vi "FindNodeAtIndex.vi"(8 "DOM document":refnum<k20>, 9 "New Node Name":string="Drive", 10 "Index":u32=13, 11 "XML String":string="\n<Sequential>\n      <Sequential>\n            <Sequential>\n                  <Hi/>\n            </Sequential>\n      </Sequential>\n      <Drive/>\n      <Sequential>\n            <Hello/>\n      </Sequential>\n</Sequential>") -> ()   [LabVIEW 2017]
uses:
  <vilib>/regexp/Match Regular Expression.xnode
  <resource>/objmgr/DOMUserDefRef.rc
  <vilib>/xml/NI_XML.lvlib
panel:
  out "XML":string
  out "submatch 1":string="Sequential"
  out "Insert as child not sibling":bool
  out "Index":i32=3
  out "Text.Selection:Start":u32=223
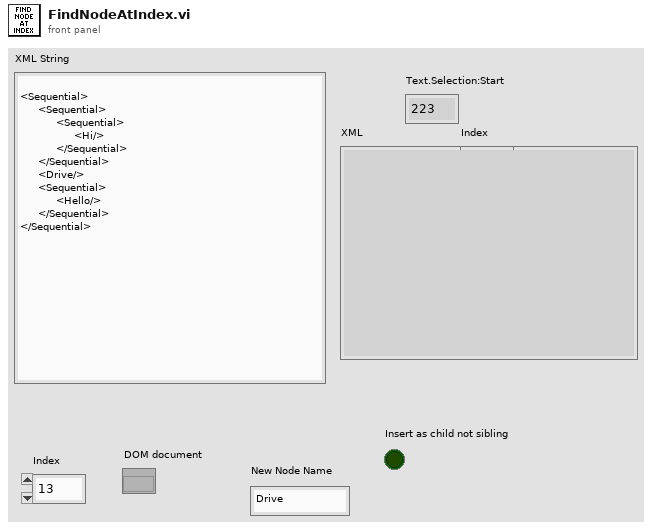
[diagram p1: front panel]
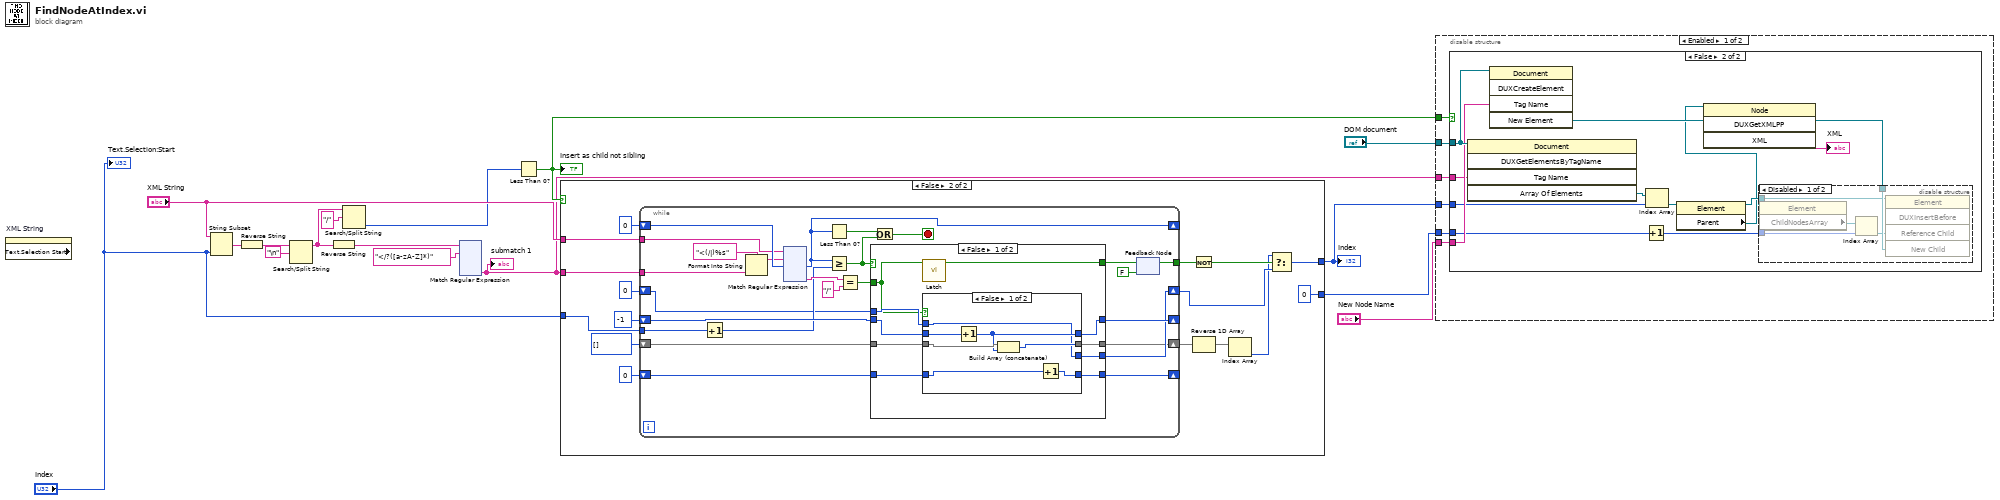
[diagram p0: block diagram]
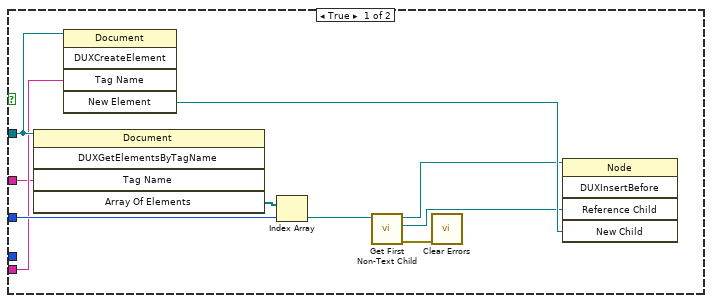
[diagram p2: hidden frame]
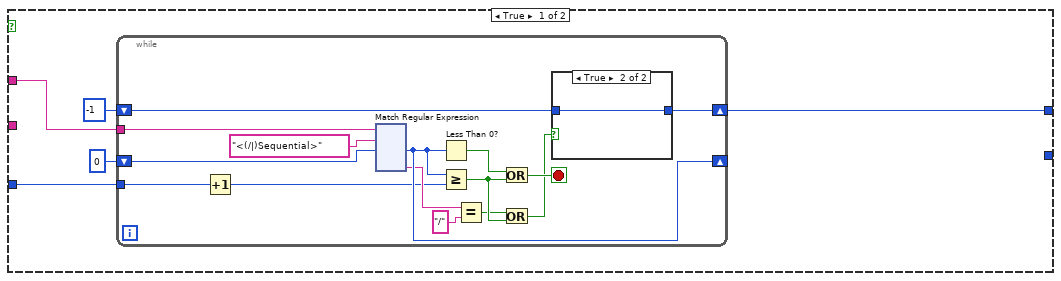
[diagram p5: hidden frame]
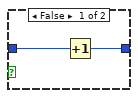
[diagram p6: hidden frame]
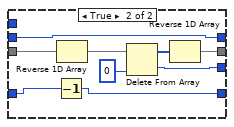
[diagram p7: hidden frame]
diagram:
  n1 = property on="XML String" class="Str" props=["Text", "Selection Start"]() -> ()  [unwired: 2 in, 3 out]
  n2 = String Subset(string="XML String", length (rest)="Index") -> (substring=w13:string)  [unwired: 1 in]
  n3 = Reverse String(1:w13) -> (0:w14:string)
  n4 = Search/Split String(string=w14, search string/char (-)="\n") -> (substring before match=w8:string)  [unwired: 1 in, 2 out]
  n5 = Reverse String(1:w8) -> (0:w10:string)
  n6 = Search/Split String(string=w8, search string/char (-)="/") -> (offset of match=w15:i32)  [unwired: 1 in, 2 out]
  n7 = xnode "Match Regular Expression"("input string"=w10, "regular expression"="</?([a-zA-Z]*)") -> ("submatch 1"=w2:string)  [unwired: 4 in, 5 out]
  "submatch 1" <- w2
  n8 = Less Than 0?(x=w15) -> (x < 0?=w5:bool)
  "Insert as child not sibling" <- w5
  n9 = case shown="False" w5 {
    tunnel: "XML String" -> [w21 w171]
    tunnel: [w18 w159] -> w7
    tunnel: "Index" -> [w17 w168]
    tunnel: [_ 0] -> w4
    tunnel: w2 -> [_ w164]
    frame True {
      n10 = while {
        tunnel: w21 -> [w26]
        shift-right: [w33] -> _
        shift-left: 0 -> [w35]
        tunnel: w17 -> [w25]
        shift-right: [w29] -> w18
        shift-left: -1 -> [w30]
        stop <- w28 stop-if-true
        n11 = Increment(x=w25) -> (x+1=w27:u32)
        n12 = xnode "Match Regular Expression"("input string"=w26, "regular expression"="<(/|)Sequential>", "offset (0)"=w35) -> ("offset past match"=w33:i32, "submatch 1"=w32:string)  [unwired: 3 in, 4 out]
        n13 = Less Than 0?(x=w33) -> (x < 0?=w34:bool)
        n14 = Greater Or Equal?(x=w33, y=w27) -> (x >= y?=w24:bool)
        n15 = Equal?(x=w32, y="/") -> (x = y?=w23:bool)
        n16 = Or(x=w34, y=w24) -> (x .or. y?=w28:bool)
        n17 = Or(x=w23, y=w24) -> (x .or. y?=w22:bool)
        n18 = case shown="True" w22 {
          tunnel: w30 -> [w37 w39]
          tunnel: [w38 w39] -> w29
          frame False {
            n19 = Increment(x=w37) -> (x+1=w38:i32)
          }
          frame True {
          }
        }
      }
    }
    frame False {
      n20 = while {
        tunnel: w171 -> [w188]
        shift-right: [w183] -> _
        shift-left: 0 -> [w196]
        tunnel: w168 -> [w187]
        shift-right: [w191] -> _
        shift-left: -1 -> [w192]
        shift-right: [w175] -> w158
        shift-left: i32[] [] -> [w182]
        shift-right: [w184] -> _
        shift-left: 0 -> [w186]
        tunnel: w164 -> [w180]
        shift-right: [w177] -> w161
        shift-left: 0 ("Numeric") -> [w176]
        tunnel: [w172] -> w162
        stop <- w190 stop-if-true
        n21 = Increment(x=w187) -> (x+1=w189:u32)
        n22 = Format Into String(format string="<(/|)%s" ("regular expression"), w180) -> (resulting string=w179:string)  [unwired: 2 in, 1 out]
        n23 = xnode "Match Regular Expression"("input string"=w188, "regular expression"=w179, "offset (0)"=w196) -> ("offset past match"=w183:i32, "submatch 1"=w194:string)  [unwired: 3 in, 4 out]
        n24 = Less Than 0?(x=w183) -> (x < 0?=w195:bool)
        n25 = Greater Or Equal?(x=w183, y=w189) -> (x >= y?=w185:bool)
        n26 = Equal?(x=w194, y="/") -> (x = y?=w178:bool)
        n27 = case shown="False" w185 {
          tunnel: w192 -> [w206 w226]
          tunnel: [w205 w226] -> w191
          tunnel: w186 -> [w204 w225]
          tunnel: w178 -> [w198 _]
          tunnel: [w199 w225] -> w184
          tunnel: w182 -> [w203 w224]
          tunnel: [w202 w224] -> w175
          tunnel: [w201 w223] -> w177
          tunnel: w176 -> [w200 w223]
          tunnel: [w197 _] -> w174
          frame False {
            n28 = call "Latch.vi"("Input"=w198) -> ("Output"=w197:bool)  [unwired: 10 in]
            n29 = case shown="False" w198 {
              tunnel: w206 -> [w211 w220]
              tunnel: [w210 w220] -> w205
              tunnel: w204 -> [w208 w215]
              tunnel: w203 -> [w213 w222]
              tunnel: [w212 w221] -> w202
              tunnel: [w209 w216] -> w201
              tunnel: w200 -> [w209 _]
              tunnel: [w207 w214] -> w199
              frame False {
                n30 = Increment(x=w211) -> (x+1=w210:i32)
                n31 = Build Array (concatenate)(w213, w210) -> (w212:i32[])
                n32 = Increment(x=w208) -> (x+1=w207:i32)
              }
              frame True {
                n33 = Decrement(x=w215) -> (x-1=w214:i32)
                n34 = Reverse 1D Array(array=w222) -> (reversed array=w219:i32[])
                n35 = Delete From Array(array=w219, index=0) -> (deleted portion=w216:i32, array with subset deleted=w217:i32[])  [unwired: 1 in]
                n36 = Reverse 1D Array(array=w217) -> (reversed array=w221:i32[])
              }
            }
          }
          frame True {
          }
        }
        n37 = Or(x=w195, y=w185) -> (x .or. y?=w190:bool)
        n38 = feedback-in #1(w174) -> ()
        n39 = feedback #1(FALSE ("Output")) -> (w172:bool)
      }
      n40 = Not(x=w162) -> (.not. x?=w160:bool)
      n41 = Reverse 1D Array(array=w158) -> (reversed array=w157:i32[])
      n42 = Index Array(array=w157) -> (element=w156:i32)  [unwired: 1 in]
      n43 = Select(t=w156, s=w160, f=w161) -> (s? t:f=w159:i32)
    }
  }
  "Index" <- w7
  n44 = disable-structure shown="Enabled" {
    disable-tunnel: "DOM document" -> [w348 _]
    disable-tunnel: w7 -> [w347 _]
    disable-tunnel: "New Node Name" -> [w346 _]
    disable-tunnel: w5 -> [w345 _]
    disable-tunnel: w2 -> [w344 _]
    disable-tunnel: w4 -> [w343 _]
    frame Enabled {
      n45 = case shown="False" w345 {
        tunnel: w348 -> [w356 w369]
        tunnel: w347 -> [w357 w364]
        tunnel: w346 -> [w355 w368]
        tunnel: w344 -> [w349 w366]
        tunnel: w343 -> [_ w362]
        frame True {
          n46 = invoke class="Document" method="DUXGetElementsByTagName"(reference=w356, "Tag Name"=w349) -> ("Array Of Elements"=w358:refnum<k20>[])  [unwired: 3 in, 4 out]
          n47 = invoke class="Document" method="DUXCreateElement"(reference=w356, "Tag Name"=w355) -> ("New Element"=w353:refnum<k20>)  [unwired: 3 in, 4 out]
          n48 = Index Array(array=w358, index=w357) -> (element=w354:refnum<k20>)
          n49 = call <vilib>:"Get First Non-Text Child.vi"("node in"=w354) -> ("error out"=w350:errorcluster, "child node"=w351:refnum<k20>, "node out"=w352:refnum<k20>)  [unwired: 7 in, 1 out]
          n50 = call <vilib>:"Clear Errors.vi"("error in (no error)"=w350) -> ()  [unwired: 5 in, 2 out]
          n51 = invoke class="Node" method="DUXInsertBefore"(reference=w352, "Reference Child"=w351, "New Child"=w353) -> ()  [unwired: 2 in, 5 out]
        }
        frame False {
          n52 = invoke class="Document" method="DUXGetElementsByTagName"(reference=w369, "Tag Name"=w366) -> ("Array Of Elements"=w370:refnum<k20>[])  [unwired: 3 in, 4 out]
          n53 = invoke class="Document" method="DUXCreateElement"(reference=w369, "Tag Name"=w368) -> ("New Element"=w367:refnum<k20>)  [unwired: 3 in, 4 out]
          n54 = Increment(x=w362) -> (x+1=w363:i32)
          n55 = Index Array(array=w370, index=w364) -> (element=w365:refnum<k20>)
          n56 = property class="Element"(reference=w365) -> (reference out=w361:refnum<k20>, "Parent"=w359:refnum<k20>)  [unwired: 1 in, 1 out]
          n57 = invoke class="Node" method="DUXGetXMLPP"(reference=w359) -> ("XML"=→"XML":string)  [unwired: 3 in, 3 out]
          n58 = disable-structure shown="Disabled" {
            disable-tunnel: w367 -> [w375 _]
            disable-tunnel: w363 -> [w373 _]
            disable-tunnel: w361 -> [w371 _]
            frame Disabled {
              n59 = property class="Element"(reference=w371) -> ("ChildNodesArray"=w374:refnum<k20>[])  [unwired: 1 in, 2 out]
              n60 = Index Array(array=w374, index=w373) -> (element=w372:refnum<k20>)
              n61 = invoke class="Element" method="DUXInsertBefore"(reference=w371, "Reference Child"=w372, "New Child"=w375) -> ()  [unwired: 2 in, 5 out]
            }
            frame Enabled {
            }
          }
        }
      }
    }
    frame Disabled {
    }
  }
  "Text.Selection:Start" <- "Index"
